vi "p2.vi"() -> ()   [LabVIEW 2021, in "d19.lvlib"]
uses:
  d19.lvlib
  Blueprint/Blueprint.lvclass
  Blueprint/Blueprint.lvclass/Blueprint.ctl
  Mine/Schedule Ore Robot.vi
  Mine/Schedule Clay Robot.vi
  Mine/Schedule Obsidian Robot.vi
  Mine/Schedule Geode Robot.vi
  Mine/Mine.lvclass
  AOC/AOC.lvlib
panel:
  out "Stack Size":i32(graph)
  in  "Force Schedule":bool
  out "Blueprint":i32=1
  in  "Forced Schedule":i32[](array[numeric])=[1, 2, 2, 2, 2, 2, 2, 2, 3, 3, 3, 3, 4, 3, 4, 4, 4, 4, 4, 4, 4, 4]
  in  "Max Time":u8=32
  out "Geodes":u8=56
  in  "Example":string="Blueprint 1:  Each ore robot costs 4 ore.  Each clay robot costs 2 ore.  Each obsidian robot costs 3 ore and 14 clay.  Each geode robot costs 2 ore and 7 obsidian.\nBlueprint 2:  Each ore robot costs 2 ore.  Each clay robot costs 3 ore.  Each obsidian robot costs 3 ore and 8 clay.  Each geode robot costs 3 ore and 12 obsidian."
  in  "Example":bool=TRUE
  out "Answer":u64=1288
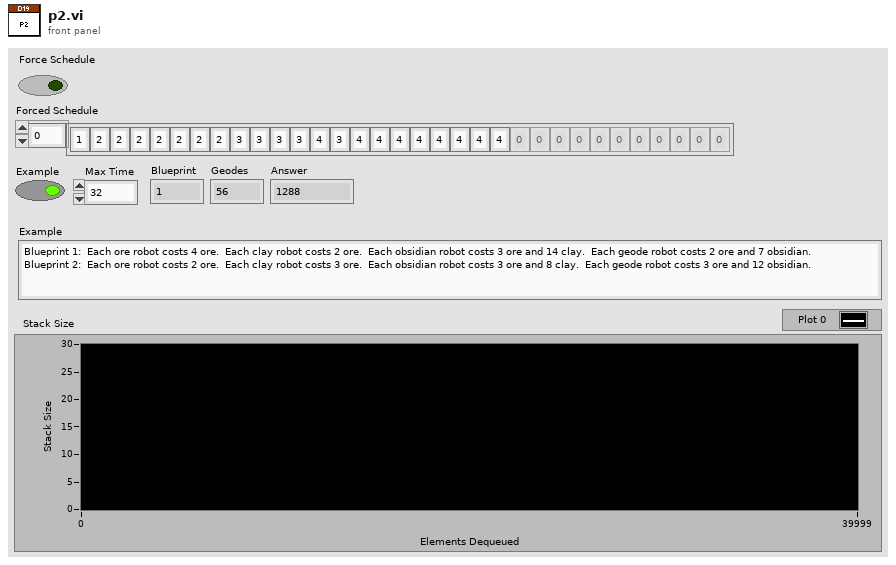
[diagram p1: front panel]
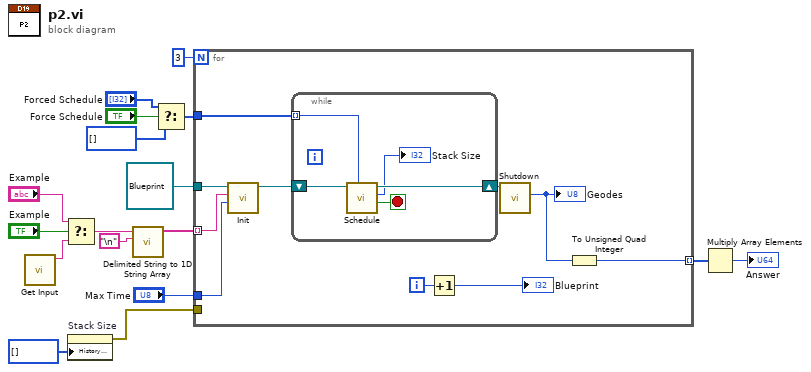
[diagram p0: block diagram]
diagram:
  n1 = call "Get Input.vi"() -> ("Input"=w17:string)  [unwired: 11 in]
  n2 = Select(t="Example", s="Example", f=w17) -> (s? t:f=w16:string)
  n3 = property on="Stack Size" class="WFChart (strict)"("History Data"=u8[] []) -> (error out=w2:errorcluster)  [unwired: 2 in, 1 out]
  n4 = call <vilib>:"Delimited String to 1D String Array.vi"("delimiter"="\n", "delimited string"=w16) -> ("string array"=w12:string[])  [unwired: 9 in]
  n5 = Select(t="Forced Schedule", s="Force Schedule", f=i32[] []) -> (s? t:f=w5:i32[])
  n6 = for {
    N: 3 -> [_]
    tunnel: w12 -> [w27] mode=indexing
    tunnel: refnum<class "Blueprint.lvclass"> refnum ("Bluepriny in") -> [w25]
    tunnel: [w20] -> w10 mode=indexing
    tunnel: "Max Time" -> [w24]
    tunnel: w5 -> [w21]
    tunnel: w2 -> [_]
    i -> [w26]
    n7 = call "Init.vi"("Max Time"=w24, "Blueprint String"=w27, "Blueprint in"=w25) -> ("Blueprint out"=w23:refnum<class "Blueprint.lvclass">)  [unwired: 8 in]
    n8 = while {
      shift-right: [w30] -> w22
      shift-left: w23 -> [w31]
      tunnel: w21 -> [w29] mode=indexing
      stop <- w32 stop-if-true
      n9 = call "Schedule.vi"("Choice"=w29, "Blueprint in"=w31) -> ("Finished?"=w32:bool, "# elements in queue"=→"Stack Size":i32, "Blueprint out"=w30:refnum<class "Blueprint.lvclass">)  [unwired: 7 in]
    }
    n10 = Increment(x=w26) -> (x+1=→"Blueprint":i32)
    n11 = call "Shutdown.vi"("Blueprint in"=w22) -> ("max geodes"=w18:u8)  [unwired: 9 in, 1 out]
    "Geodes" <- w18
    n12 = To Unsigned Quad Integer(1:w18) -> (0:w20:u64)
  }
  n13 = Multiply Array Elements(1:w10) -> (0:→"Answer":u64)
